vi "Edgepoints2Polypoints.vi"(8 "Scaling Factor":dbl, 10 "Edgepoints In":cluster{"Row":i32, "Col":i32}[][](array[cluster])) -> (3 "Polyline Out":dbl[][][](array[numeric]))   [LabVIEW 2019]
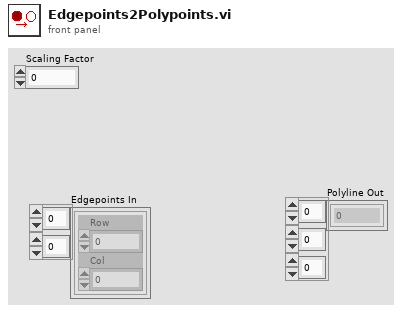
[diagram p1: front panel]
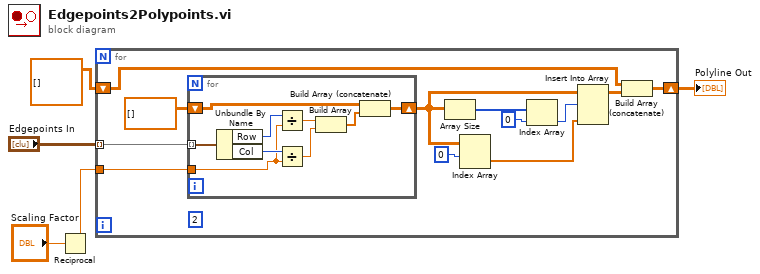
[diagram p0: block diagram]
diagram:
  n1 = Reciprocal(x="Scaling Factor") -> (1/x=w2:dbl)
  n2 = for {
    tunnel: "Edgepoints In" -> [w17] mode=indexing
    shift-right: [w16] -> w5
    shift-left: dbl[][][] [] ("Array in") -> [w15]
    tunnel: w2 -> [w6]
    (unwired) 2 ("index (row)")
    n3 = for {
      tunnel: w17 -> [w26] mode=indexing
      shift-right: [w25] -> w10
      shift-left: dbl[][] [] -> [w23]
      tunnel: w6 -> [w18]
      n4 = Unbundle By Name(w26) -> ("Row"=w22:i32, "Col"=w21:i32)
      n5 = Divide(x=w22, y=w18) -> (x/y=w20:dbl)
      n6 = Divide(x=w21, y=w18) -> (x/y=w19:dbl)
      n7 = Build Array(w20, w19) -> (w24:dbl[])
      n8 = Build Array (concatenate)(w23, w24) -> (w25:dbl[][])
    }
    n9 = Array Size(array=w10) -> (size(s)=w9:i32[])
    n10 = Index Array(array=w10, index (row)=0) -> (element=w12:dbl[])  [unwired: 1 in]
    n11 = Index Array(array=w9, index=0) -> (element=w7:i32)
    n12 = Insert Into Array(array=w10, index (row)=w7, new element=w12) -> (w11:dbl[][])  [unwired: 1 in]
    n13 = Build Array (concatenate)(w15, w11) -> (w16:dbl[][][])
  }
  "Polyline Out" <- w5
